vi "SourceDequeueLatestCommand.vi"(3 "Queue in":refnum<queue>, 9 "error in (no error)":errorcluster) -> (0 "Queue out":refnum<queue>, 2 "SourceCommand":T1, 6 "error out":errorcluster)   [LabVIEW 2009]
uses:
  Controls/SourceCommand.ctl
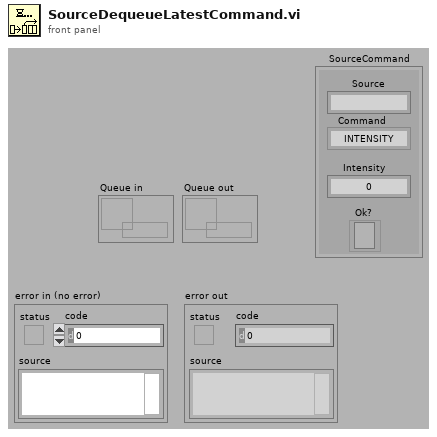
[diagram p1: front panel]
types:
  T1 = typedef "SourceCommand.ctl" = cluster{"Source":string, "Command":enum16{"INTENSITY", "ALL OFF", "QUIT"}, "Intensity":i32, "Ok?":refnum<k4>}
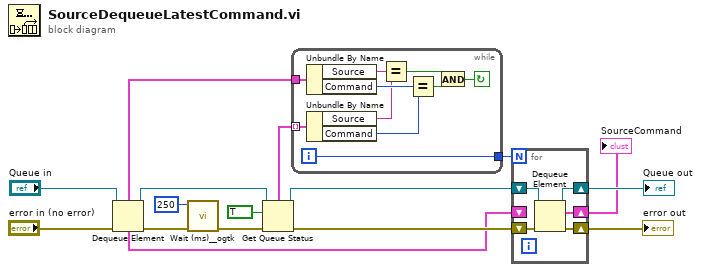
[diagram p0: block diagram]
diagram:
  n1 = Dequeue Element(queue="Queue in", error in (no error)="error in (no error)") -> (queue out=w8:refnum<queue>, element=w2:T1, error out=w12:errorcluster)  [unwired: 2 out]
  n2 = call <userlib>:"Wait (ms)__ogtk.vi"("error in (no error)"=w12, "milliseconds to wait"=u32 250) -> ("error out"=w13:errorcluster)  [unwired: 1 in, 8 out]
  n3 = Get Queue Status(queue=w8, return elements? (F)=TRUE, error in (no error)=w13) -> (queue out=w7:refnum<queue>, error out=w9:errorcluster, elements=w4:T1[])  [unwired: 5 out]
  n4 = while {
    tunnel: [w21] -> w3
    tunnel: w2 -> [w19]
    tunnel: w4 -> [w18] mode=indexing
    i -> [w21]
    stop <- w20 continue-if-true
    n5 = Unbundle By Name(w19) -> ("Source"=w25:string, "Command"=w24:enum16{"INTENSITY", "ALL OFF", "QUIT"})
    n6 = Unbundle By Name(w18) -> ("Source"=w17:string, "Command"=w16:enum16{"INTENSITY", "ALL OFF", "QUIT"})
    n7 = Equal?(x=w25, y=w17) -> (x = y?=w23:bool)
    n8 = Equal?(x=w24, y=w16) -> (x = y?=w22:bool)
    n9 = And(x=w23, y=w22) -> (x .and. y?=w20:bool)
  }
  n10 = for {
    N: w3 -> [_]
    shift-right: [w27] -> w6
    shift-left: w7 -> [w28]
    shift-right: [w26] -> w5
    shift-left: w9 -> [w30]
    shift-right: [w29] -> w1
    shift-left: w2 -> [_]
    n11 = Dequeue Element(queue=w28, error in (no error)=w30) -> (queue out=w27:refnum<queue>, element=w29:T1, error out=w26:errorcluster)  [unwired: 2 out]
  }
  "Queue out" <- w6
  "error out" <- w5
  "SourceCommand" <- w1
